vi "Inspect - Get Inspection Status.vi"(8 "error in (no error)":errorcluster) -> (0 "error out":errorcluster, 3 "Inspection Status":bool)   [LabVIEW 2019]
uses:
  Common.llb/IVB Measure ID.ctl
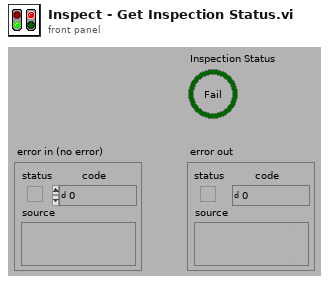
[diagram p1: front panel]
types:
  T1 = typedef "IVB Measure ID.ctl" = cluster{"Step GUID":string, "Result GUID":string, "Index":i32}
  T2 = cluster{"Numeric":dbl, "Boolean":bool, "String":string, "1D Numeric":dbl[], "1D Boolean":bool[], "1D String":string[]}
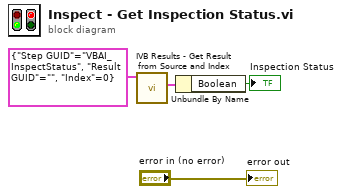
[diagram p0: block diagram]
diagram:
  n1 = call "IVB Results - Get Result from Source and Index.vi"("Measure ID"=T1 {"Step GUID"="VBAI_InspectStatus", "Result GUID"="", "Index"=0}) -> ("Result Value"=w1:T2)  [unwired: 6 in, 4 out]
  n2 = Unbundle By Name(w1) -> ("Boolean"=→"Inspection Status":bool)
  "error out" <- "error in (no error)"
